vi "save_dictionary.vi"   [LabVIEW 2015, in "lv-unit-conversion.lvlib"]
uses:
  lv-unit-conversion.lvlib
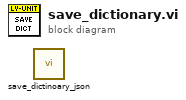
[diagram p0: block diagram]
diagram:
  n1 = call "save_dictinoary_json.vi"() -> ()  [unwired: 11 in, 1 out]
